vi "MRCMDFBGlobal.vi"() -> ()   [LabVIEW 2016]
uses:
  CorrectionsCluster.ctl
  SingleMeas_Repeater.ctl
  ProfCoords.ctl
  MRBRowTaskSelector.ctl
panel:
  in  "Tab Control":T1(tab)
  in  "What Rig is\nMultirunning?":string="WT3"
  in  "Jump Bad Positions":bool
  in  "Work in TUNNEL Coordinates":bool
  in  "Setup:":string="Pitot_5HP.xls"
  in  "Command File Path / Name":path=path "AnemometerSurvey.xls"
  in  "Results File Path / Name":path=path "AnemometerSurvey.xls"
  in  "Tunnel Warmup (min)":dbl=30.0
  in  "Velocity (m/s)":dbl=10.75
  in  "Measure (seconds)":dbl=60.0
  in  "Task Selection":T2={"Tunnel Warm Up"=TRUE, "AutoCal"=FALSE, "Zeroes 2"=TRUE, "Turn Table Schedule"=TRUE, "Global Cal Checks"=TRUE, "Local Cal Checks"=TRUE, "Vertical Profile"=TRUE, "Lateral Profile"=FALSE, "Reinitialize Task Array"=TRUE, "Save Command File"=TRUE, "Longitudinal Profile"=FALSE}
  in  "Multirun Closure Tasks":T3={"Tunnel Off"=TRUE, "Local Cal Checks"=TRUE, "Global Cal Checks"=TRUE, "Zeroes"=TRUE, "AutoCal"=FALSE, "Turn Table --> Zero"=TRUE}
  in  "SingleMeasurement.Coords":T4(array[cluster])
  in  "Zeroes":T5={"X"=-3390.0, "Y"=-113.0, "Z"=900.0, "Use Tunnel Coords?"=TRUE, "RepeatEveryXDeg"=120.0}
  in  "Local Calcheck":T5={"X"=0.0, "Y"=0.0, "Z"=900.0, "Use Tunnel Coords?"=TRUE, "RepeatEveryXDeg"=60.0}
  in  "Global Calcheck":T5={"X"=-3390.0, "Y"=-113.0, "Z"=900.0, "Use Tunnel Coords?"=TRUE, "RepeatEveryXDeg"=120.0}
  in  "Calculate TT Array":bool=TRUE
  in  "Angle Increment":dbl=20.0
  in  "Ending Angle":dbl=360.0
  in  "Starting Angle":dbl
  in  "Azimuth Values":dbl[](array[numeric])
  in  "Build-A-Block":T7(array[cluster])
  in  "VertProf.Coords":T8
  in  "VP.TTHeightCorrs":T9={"Use Height Corrections"=FALSE, "TT.Azimuths"=[], "Z.HeightCorrs"=[], "Corrections from File"=TRUE, "Height Survey Filepaths"=[]}
  in  "Correction Channel Name":string
  in  "LatProf.Coords":T8
  in  "Lat.HeightCorrs":T9={"Use Height Corrections"=TRUE, "TT.Azimuths"=[0.0], "Z.HeightCorrs"=[], "Corrections from File"=TRUE, "Height Survey Filepaths"=[]}
  in  "LongProf.Coords":T8
  in  "Long.HeightCorrs":T9={"Use Height Corrections"=TRUE, "TT.Azimuths"=[0.0], "Z.HeightCorrs"=[], "Corrections from File"=TRUE, "Height Survey Filepaths"=[]}
  in  "MoveTrav.Coords":T10(array[cluster])
  in  "Autocal.TunnelSpeeds":dbl[](array[numeric])
  in  "SpeedSettings":dbl[](array[numeric])
  in  "Wait Time (min)":dbl[](array[numeric])=[1440.0]
  in  "MessagesArray":string[](array[string])=["Time to set the ramps..."]
  out "Audit Array":string[](array[string])=["Initialize", "Build TT Array", "Warm Up", "Zeroes", "AutoCal", "GlobalCalCheck", "LocalCalCheck", "Turn Table Schedule", "Vertical Corrections", "Vertical Profile", "Vertical Corrections", "Vertical Profile", "Lateral Profile", "Longitudinal Profile", "Repeat?", "Zeroes", "AutoCal", "GlobalCalCheck", "LocalCalCheck", "Turn Table Schedule", "Vertical Corrections", "Vertical Profile", "Vertical Corrections", "Vertical Profile", "Lateral Profile", "Longitudinal Profile", "Repeat?", "Zeroes", "AutoCal", "GlobalCalCheck", "LocalCalCheck", "Turn Table Schedule", "Vertical Corrections", "Vertical Profile", "Vertical Corrections", "Vertical Profile", "Lateral Profile", "Longitudinal Profile", "Repeat?", "Zeroes", "AutoCal", "GlobalCalCheck", "LocalCalCheck", "Turn Table Schedule", "Vertical Corrections", "Vertical Profile", "Vertical Corrections", "Vertical Profile", "Lateral Profile", "Longitudinal Profile", "Repeat?", "Zeroes", "AutoCal", "GlobalCalCheck", "LocalCalCheck", "Turn Table Schedule", "Vertical Corrections", "Vertical Profile", "Vertical Corrections", "Vertical Profile", "Lateral Profile", "Longitudinal Profile", "Repeat?", "Zeroes", "AutoCal", "GlobalCalCheck", "LocalCalCheck", "Turn Table Schedule", "Vertical Corrections", "Vertical Profile", "Vertical Corrections", "Vertical Profile", "Lateral Profile", "Longitudinal Profile", "Repeat?", "Zeroes", "AutoCal", "GlobalCalCheck", "LocalCalCheck", "Turn Table Schedule", "Vertical Corrections", "Vertical Profile", "Vertical Corrections", "Vertical Profile", "Lateral Profile", "Longitudinal Profile", "Repeat?", "Zeroes", "AutoCal", "GlobalCalCheck", "LocalCalCheck", "Turn Table Schedule", "Vertical Corrections", "Vertical Profile", "Vertical Corrections", "Vertical Profile", "Lateral Profile", "Longitudinal Profile", "Repeat?", "Zeroes", "AutoCal", "GlobalCalCheck", "LocalCalCheck", "Turn Table Schedule", "Vertical Corrections", "Vertical Profile", "Vertical Corrections", "Vertical Profile", "Lateral Profile", "Longitudinal Profile", "Repeat?", "Zeroes", "AutoCal", "GlobalCalCheck", "LocalCalCheck", "Turn Table Schedule", "Vertical Corrections", "Vertical Profile", "Vertical Corrections", "Vertical Profile", "Lateral Profile", "Longitudinal Profile", "Repeat?", "Zeroes", "AutoCal", "GlobalCalCheck", "LocalCalCheck", "Turn Table Schedule", "Vertical Corrections", "Vertical Profile", "Vertical Corrections", "Vertical Profile", "Lateral Profile", "Longitudinal Profile", "Repeat?", "Zeroes", "AutoCal", "GlobalCalCheck", "LocalCalCheck", "Turn Table Schedule", "Vertical Corrections", "Vertical Profile", "Vertical Corrections", "Vertical Profile", "Lateral Profile", "Longitudinal Profile", "Repeat?", "Zeroes", "AutoCal", "GlobalCalCheck", "LocalCalCheck", "Turn Table Schedule", "Vertical Corrections", "Vertical Profile", "Vertical Corrections", "Vertical Profile", "Lateral Profile", "Longitudinal Profile", "Repeat?", "Zeroes", "AutoCal", "GlobalCalCheck", "LocalCalCheck", "Turn Table Schedule", "Vertical Corrections", "Vertical Profile", "Vertical Corrections", "Vertical Profile", "Lateral Profile", "Longitudinal Profile", "Repeat?", "Zeroes", "AutoCal", "GlobalCalCheck", "LocalCalCheck", "Turn Table Schedule", "Vertical Corrections", "Vertical Profile", "Vertical Corrections", "Vertical Profile", "Lateral Profile", "Longitudinal Profile", "Repeat?", "Zeroes", "AutoCal", "GlobalCalCheck", "LocalCalCheck", "Turn Table Schedule", "Vertical Corrections", "Vertical Profile", "Vertical Corrections", "Vertical Profile", "Lateral Profile", "Longitudinal Profile", "Repeat?", "Zeroes", "AutoCal", "GlobalCalCheck", "LocalCalCheck", "Turn Table Schedule", "Vertical Corrections", "Vertical Profile", "Vertical Corrections", "Vertical Profile", "Lateral Profile", "Longitudinal Profile", "Repeat?", "Zeroes", "AutoCal", "GlobalCalCheck", "LocalCalCheck", "Turn Table Schedule", "Vertical Corrections", "Vertical Profile", "Vertical Corrections", "Vertical Profile", "Lateral Profile", "Longitudinal Profile", "Repeat?", "End"]
  in  "Index Tracking":T11
  out "Measure (mins)":dbl=1.0
  # "#ToDo Add the bit that was used to gen\nflight path survey"
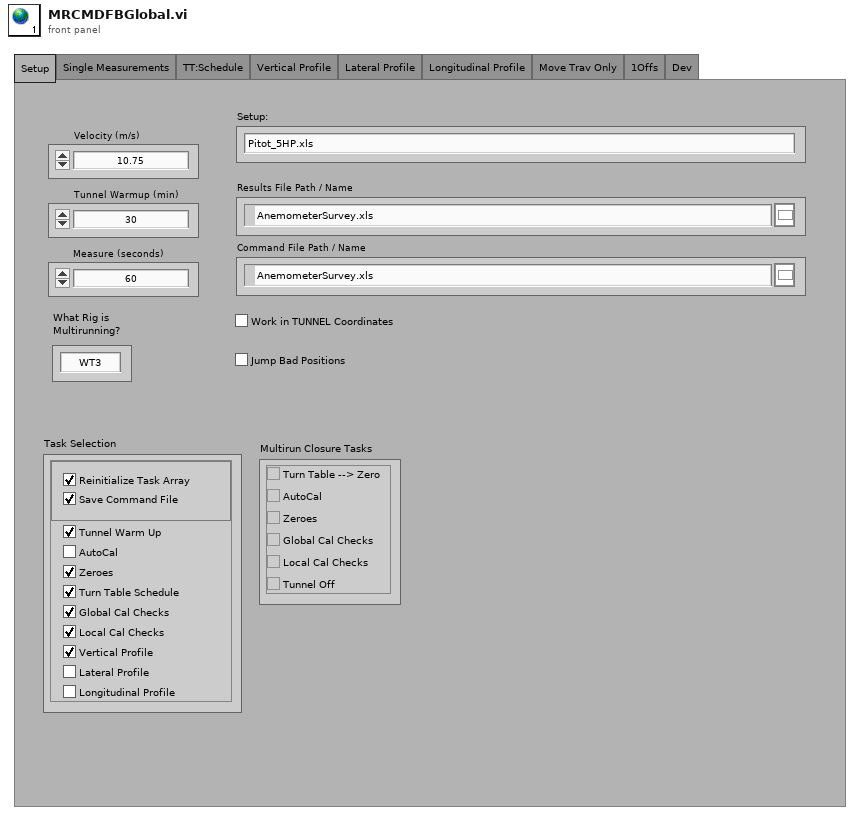
[diagram p1: front panel]
types:
  T1 = enum32{"Setup", "Single Measurements", "TT:Schedule", "Vertical Profile", "Lateral Profile", "Longitudinal Profile", "Move Trav Only", "1Offs", "Dev"}
  T2 = cluster{"Tunnel Warm Up":bool, "AutoCal":bool, "Zeroes 2":bool, "Turn Table Schedule":bool, "Global Cal Checks":bool, "Local Cal Checks":bool, "Vertical Profile":bool, "Lateral Profile":bool, "Reinitialize Task Array":bool, "Save Command File":bool, "Longitudinal Profile":bool}
  T3 = cluster{"Tunnel Off":bool, "Local Cal Checks":bool, "Global Cal Checks":bool, "Zeroes":bool, "AutoCal":bool, "Turn Table --> Zero":bool}
  T4 = cluster{"X":dbl, "Y":dbl, "Z":dbl, "Name":string, "Use Tunnel Coords?":bool}[]
  T5 = typedef "SingleMeas_Repeater.ctl" = cluster{"X":dbl, "Y":dbl, "Z":dbl, "Use Tunnel Coords?":bool, "RepeatEveryXDeg":dbl}
  T6 = typedef "MRBRowTaskSelector.ctl" = enum16{"Move Traverse Only", "Set Tunnel Speed Only", "Set Source Only", "Set Measurement Conditions", "Single Measurement", "Vertical Profile", "Lateral Profile", "Longitudinal Profile", "Explore Volume", "Multi-Axis Profile", "Auto Calibrate", "Meas Fast FID Bkgnd", "Check Beam Power", "Scanning Valve Measurement", "Run VI Named:", "MoveTT", "TravZSurvey", "Set ADAM Ch", "Wait (minutes)", "Send Message", "Synchronize With:", "Fall Back to this Row", "Turn Off Row Repeating", "Blank Row", "Traverse 3D Volume"}
  T7 = cluster{"Row Type Selector":T6, "Index":dbl, "Direction":enum16{"Forward", "Reverse"}}[]
  T8 = typedef "ProfCoords.ctl" = cluster{"X":dbl, "Y":dbl, "Z":dbl, "Name":string, "Spacing":enum16{"Linear", "Log", "Gauss", "Specified", "N/A"}, "start":dbl, "end":dbl, "NumPts":dbl, "Specified Locns":dbl[]}[]
  T9 = typedef "CorrectionsCluster.ctl" = cluster{"Use Height Corrections":bool, "TT.Azimuths":dbl[], "Z.HeightCorrs":dbl[][], "Corrections from File":bool, "Height Survey Filepaths":path[]}
  T10 = cluster{"X":dbl, "Y":dbl, "Z":dbl, "Comment":string, "Use Tunnel Coords?":bool}[]
  T11 = cluster{"Azimuth Array Index":u32, "Vert Prof Array Index":u32, "Lat Prof Array Index":u32, "Long Prof Array Index":u32}
diagram:
